vi "Shoot Cube Requested.vi"(9 "Other Command Requested?":bool, 10 "Stored Game Piece":T1, 11 "Driver Buttons":bool[](array[boolean])) -> (2 "Shoot Cube Pressed?":bool, 3 "Shoot Cube Requested?":bool)   [LabVIEW 2020]
uses:
  manipulator/Implementation/Typedefs/game object.ctl
  <vilib>/Rock Robotics/WPI/Joystick/XBox Buttons Indexer.ctl
  67ce35ec-8c60-4e19-863b-667b20b85013.vi
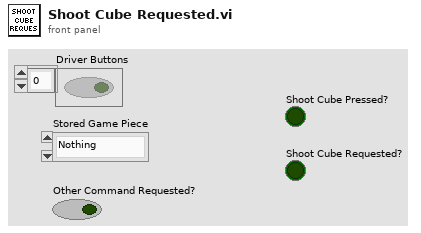
[diagram p1: front panel]
types:
  T1 = typedef "game object.ctl" = enum16{"Nothing", "Cone", "Cube"}
  T2 = typedef "XBox Buttons Indexer.ctl" = enum16{"A", "B", "X", "Y", "Left Bumper", "Right Bumper", "Back", "Start", "Left Joystick", "Right Joystick"}
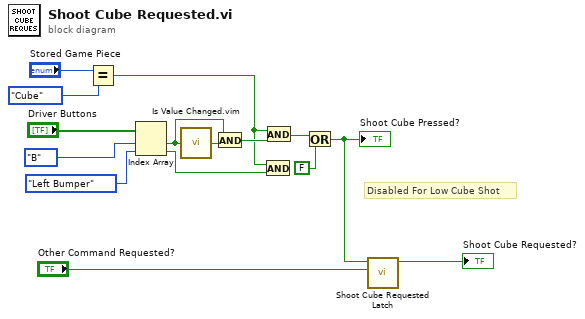
[diagram p0: block diagram]
diagram:
  # "Disabled For Low Cube Shot"
  n1 = Equal?(x="Stored Game Piece", y=game_object."Cube") -> (x = y?=w4:bool)
  n2 = Index Array(array="Driver Buttons", index #1=XBox_Buttons_Indexer."B" ("XBox Buttons"), index #2=XBox_Buttons_Indexer."Left Bumper" ("XBox Buttons")) -> (element #1=w12:bool, element #2=w5:bool)
  n3 = call "Is Value Changed.vim"("value"=w12) -> ("changed or first call?"=w13:bool)
  n4 = And(x=w12, y=w13) -> (x .and. y?=w9:bool)
  n5 = And(x=w4, y=w5) -> ()  [unwired: 1 out]
  n6 = And(x=w4, y=w9) -> (x .and. y?=w3:bool)
  n7 = Or(x=w3, y=FALSE) -> (x .or. y?=w2:bool)
  "Shoot Cube Pressed?" <- w2
  n8 = call "Shoot Cube Requested Latch.vi"("Other Command Requested?"="Other Command Requested?", "Shoot Cube Pressed?"=w2) -> ("Shoot Cube Requested?"=→"Shoot Cube Requested?":bool)  [unwired: 9 in]
